vi "lua_tolstring.vi"(8 "error in (no error)":errorcluster, 10 "index":i32, 11 "lua_state_p":u64) -> (0 "error out":errorcluster, 2 "string":string, 3 "lua_state_p out":u64)   [LabVIEW 2020, in "lua.dll.lvlib"]
doc: "lua_tolstring\n[-0, +0, m]\nconst char *lua_tolstring (lua_State *L, int index, size_t *len);\nConverts the Lua value at the given index to a C string. If len is not NULL, it sets *len with the string length. The Lua value must be a string or a number; otherwise, the function returns NULL. If the value is a number, then lua_tolstring also changes the actual value in the stack to a string. (This change confuses lua_next when lua_tolstring is applied to keys during a table traversal.)\n\nlua_tolstring returns a pointer to a string inside the Lua state. This string always has a zero ('\\0') after its last character (as in C), but can contain other zeros in its body.\n\nBecause Lua has garbage collection, there is no guarantee that the pointer returned by lua_tolstring will be valid after the corresponding Lua value is removed from the stack."
uses:
  lua.dll.lvlib
  lua54.dll
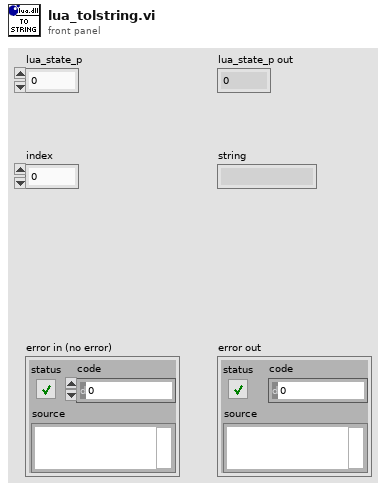
[diagram p1: front panel]
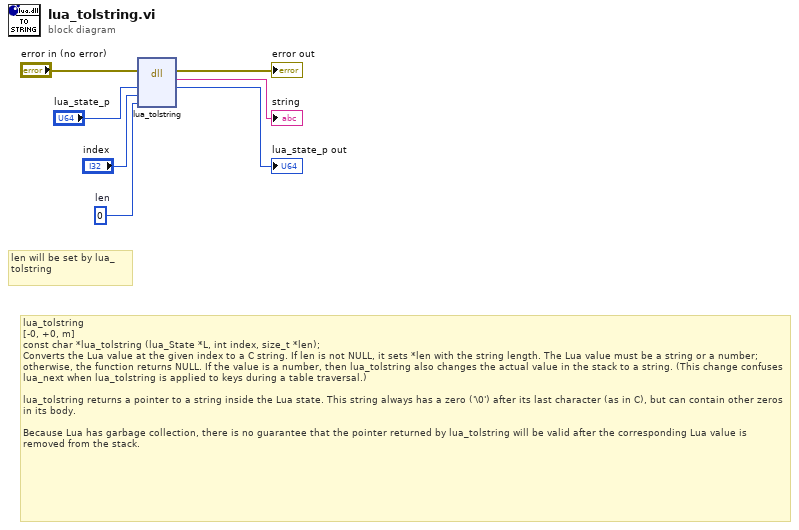
[diagram p0: block diagram]
diagram:
  w4 = u64 0  # len
  # "len will be set by lua_tolstring"
  # "lua_tolstring\n[-0, +0, m]\nconst char *lua_tolstring (lua_State *L, int index, size_t *len);\nConverts the Lua value at the given index to a C string. If len is not NULL, it sets *len with the string length. The Lua value must be a string or a number; otherwise, the function returns NULL. If the value is a number, then lua_tolstring also changes the actual value in the stack to a string. (This change confuses lua_next when lua_tolstring is applied to keys during a table traversal.)\n\nlua_tolstring returns a pointer to a string inside the Lua state. This string always has a zero ('\\0') after its last character (as in C), but can contain other zeros in its body.\n\nBecause Lua has garbage collection, there is no guarantee that the pointer returned by lua_tolstring will be valid after the corresponding Lua value is removed from the stack."
  n1 = dll-call lib="C:/Users/Nicholas Folse/Documents/workspace/github-tauterra.llc/Lua for LabVIEW/lib/lua.dll/lua54**.*" fn="lua_tolstring"(error in="error in (no error)", "lua_state_p"="lua_state_p", "index"="index", "len"=w4) -> (error out=→"error out":errorcluster, "result"=→"string":string, "lua_state_p"=→"lua_state_p out":u64)  [unwired: 4 in, 1 out]
